vi "Do Transition.vi"(5 "VolatusAPI":refnum<class "VolatusAPI.lvclass">, 6 "State Loop Data in":T1, 7 "State Control":T9, 9 "Seq Name":string, 10 "Met Conditions":refnum<class "Condition.lvclass">[](array[class]), 11 "State in":refnum<class "State.lvclass">) -> (3 "State out":refnum<class "State.lvclass">, 4 "State Loop Data":T1)   [LabVIEW 2023, in "VolatusSeq.lvlib" / "State.lvclass"]
uses:
  State.lvclass
  State Control.ctl
  Sequence Time.ctl
  Variables/Variables.lvclass
  State Loop Data.ctl
  Iteration Actions/Iteration Actions.lvclass
  Command.ctl
  VolatusSeqConfig/Command Type.ctl
  messages/CmdDigital/Data.ctl
  messages/CmdAnalog/Data.ctl
  Send Type.ctl
  Volatus/VolatusAPI/VolatusAPI.lvclass
  Condition/Condition.lvclass
  Iteration Actions/Iteration Actions.lvclass/Iteration Actions.ctl
  State.lvclass/State.ctl
  VolatusSeq.lvlib
  Transition/Transition.lvclass
  VolatusSeqConfig/VolatusSeqConfig.lvlib
  Volatus/MessageQ/MessageQ.lvclass
  messages/CmdDigital/CmdDigital.lvlib
  messages/CmdAnalog/CmdAnalog.lvlib
  lv-vecto/Vecto/Channel DBL/Channel DBL.lvclass
  Format String/Format String.lvclass
  VolatusSeqConfig/Debug Flags.ctl
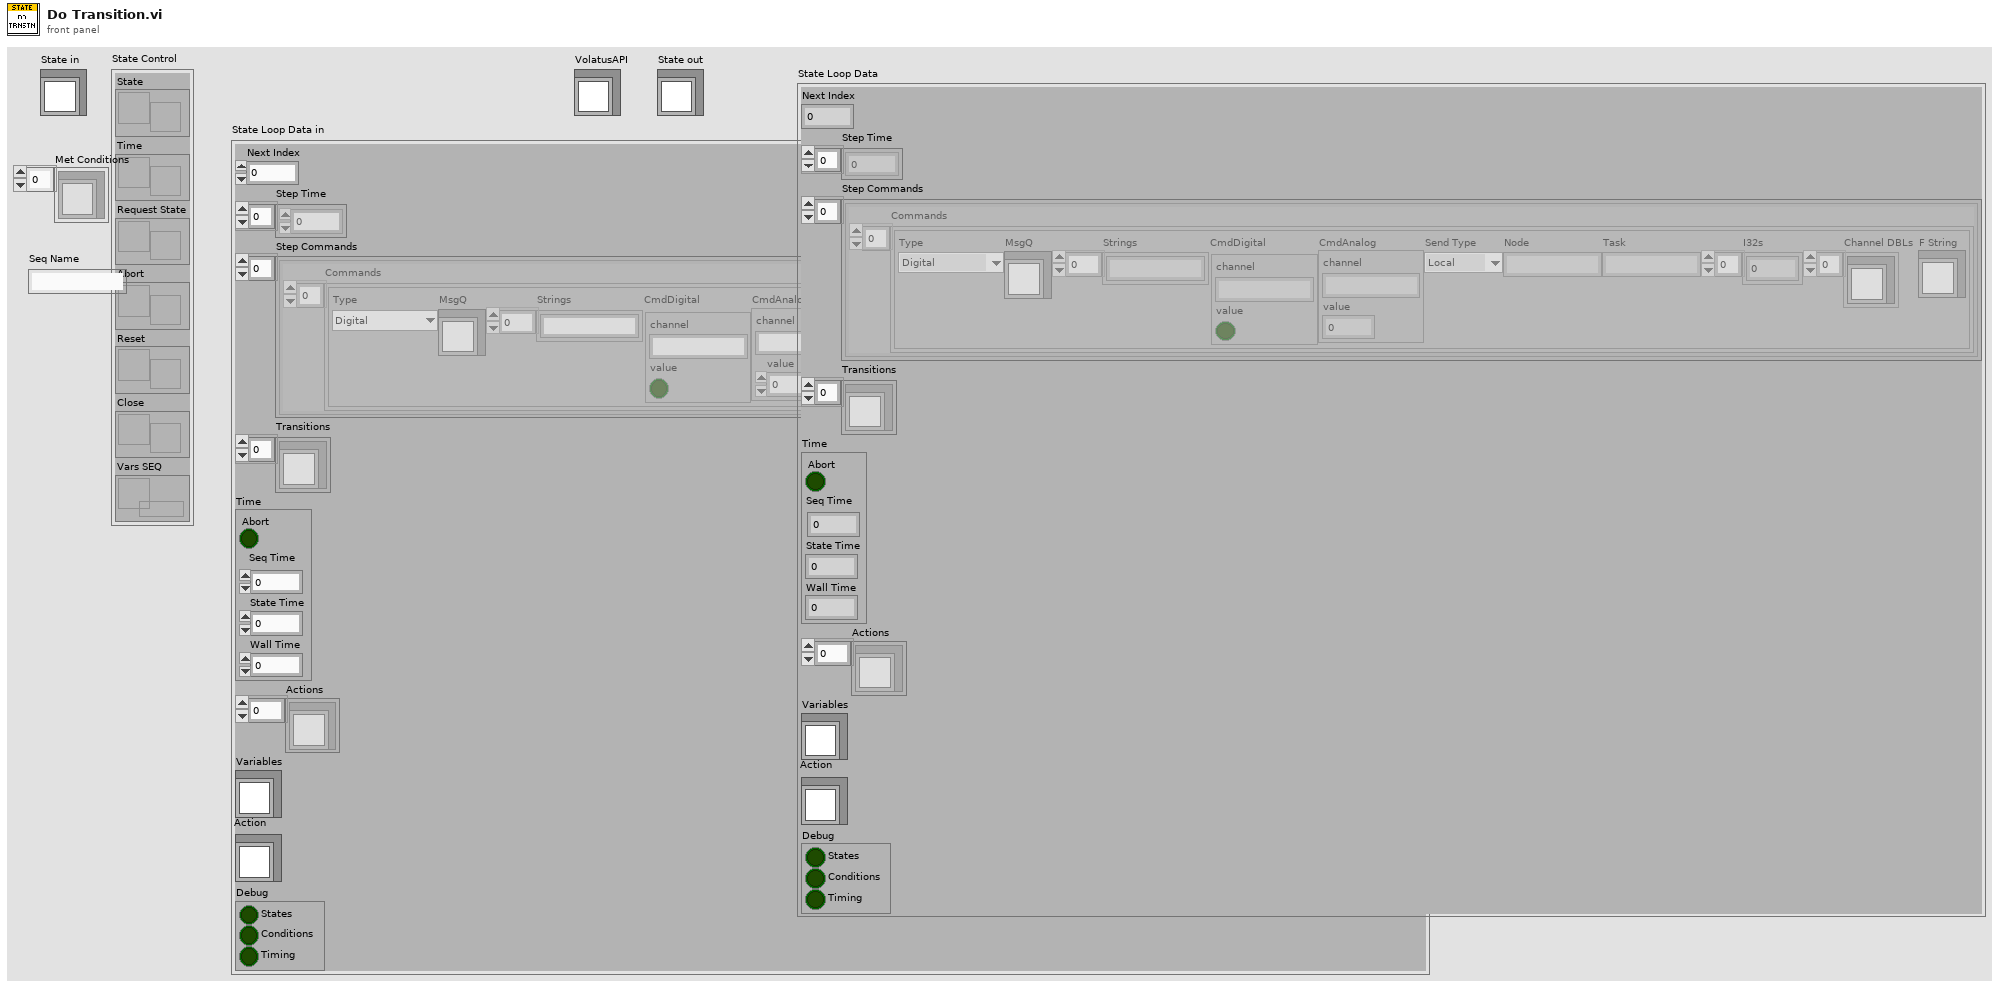
[diagram p1: front panel]
types:
  T1 = typedef "VolatusSeq.lvlib/State.lvclass/State Loop Data.ctl" = cluster{"Next Index":i32, "Step Time":dbl[], "Step Commands":cluster{"Commands":T2[]}[], "Transitions":refnum<class "Transition.lvclass">[], "Time":T7, "Actions":refnum<class "Iteration Actions.lvclass">[], "Variables":refnum<class "Variables.lvclass">, "Action":refnum<class "Iteration Actions.lvclass">, "Debug":T8}
  T2 = typedef "VolatusSeq.lvlib/Command.ctl" = cluster{"Type":T3, "MsgQ":refnum<class "MessageQ.lvclass">, "Strings":string[], "CmdDigital":T4, "CmdAnalog":T5, "Send Type":T6, "Node":string, "Task":string, "I32s":i32[], "Channel DBLs":refnum<class "Channel DBL.lvclass">[], "F String":refnum<class "Format String.lvclass">}
  T3 = typedef "VolatusSeqConfig.lvlib/Command Type.ctl" = enum16{"Digital", "Numeric", "Transition", "Stop", "StartLog", "StopLog", "Start", "Event", "Error", "HTTP", "ResetVar", "IncVar", "DecVar", "SaveVar", "LoadVar", "AddVar", "SubVar", "SetVar", "AddToVar"}
  T4 = typedef "CmdDigital.lvlib/Data.ctl" = cluster{"channel":string, "value":bool}
  T5 = typedef "CmdAnalog.lvlib/Data.ctl" = cluster{"channel":string, "value":dbl}
  T6 = typedef "VolatusSeq.lvlib/Send Type.ctl" = enum16{"Local", "Remote"}
  T7 = typedef "VolatusSeq.lvlib/Sequence Time.ctl" = cluster{"Abort":bool, "Seq Time":dbl, "State Time":dbl, "Wall Time":dbl}
  T8 = typedef "VolatusSeqConfig.lvlib/Debug Flags.ctl" = cluster{"States":bool, "Conditions":bool, "Timing":bool}
  T9 = typedef "VolatusSeq.lvlib/State Control.ctl" = cluster{"State":refnum<notifier>, "Time":refnum<notifier>, "Request State":refnum<notifier>, "Abort":refnum<notifier>, "Reset":refnum<notifier>, "Close":refnum<notifier>, "Vars SEQ":refnum<queue>}
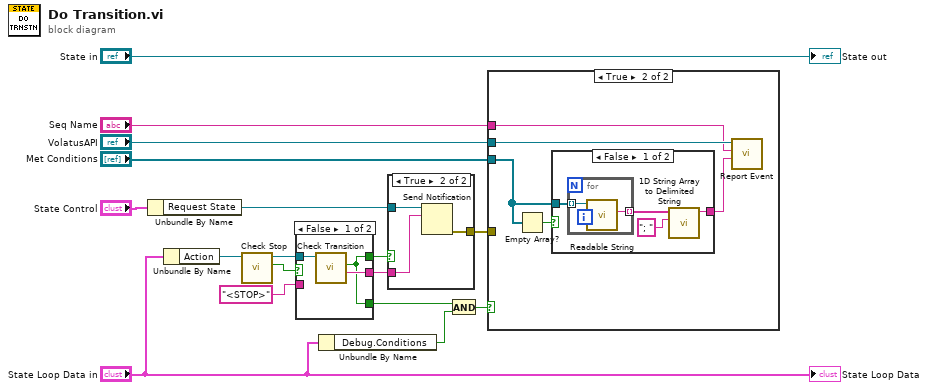
[diagram p0: block diagram]
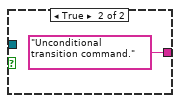
[diagram p3: hidden frame]
diagram:
  n1 = Unbundle By Name("State Control") -> ("Request State"=w13:refnum<notifier>)
  n2 = Unbundle By Name("State Loop Data in") -> ("Action"=w16:refnum<class "Iteration Actions.lvclass">)
  n3 = call "Check Stop.vi"("Iteration Actions in"=w16) -> ("Stop Seq"=w11:bool, "Iteration Actions out"=w12:refnum<class "Iteration Actions.lvclass">)  [unwired: 8 in, 1 out]
  n4 = case shown="False" w11 {
    selector: w11 -> [_ w22]
    tunnel: [w18 w22] -> w15
    tunnel: [w20 w21] -> w10
    tunnel: w12 -> [w19 _]
    tunnel: "<STOP>" ("Next State") -> [_ w21]
    tunnel: [w18 _] -> w7
    frame False {
      n5 = call "Check Transition.vi"("Iteration Actions in"=w19) -> ("Next State"=w20:string, "Transition"=w18:bool)  [unwired: 7 in, 2 out]
    }
    frame True {
    }
  }
  n6 = Unbundle By Name("State Loop Data in") -> ("Debug.Conditions"=w6:bool)
  n7 = case shown="True" w15 {
    tunnel: w10 -> [_ w24]
    tunnel: w13 -> [_ w25]
    tunnel: [_ w23] -> w2
    frame False {
    }
    frame True {
      n8 = Send Notification(notification=w24, notifier=w25) -> (error out=w23:errorcluster)  [unwired: 1 in, 1 out]
    }
  }
  n9 = And(x=w7, y=w6) -> (x .and. y?=w5:bool)
  n10 = case shown="True" w5 {
    tunnel: "VolatusAPI" -> [_ w30]
    tunnel: "Seq Name" -> [_ w29]
    tunnel: "Met Conditions" -> [_ w27]
    tunnel: w2 -> [_ _]
    frame False {
    }
    frame True {
      n11 = Empty Array?(array=w27) -> (empty?=w26:bool)
      n12 = case shown="False" w26 {
        tunnel: [w32 "Unconditional transition command." ("delimited string")] -> w28
        tunnel: w27 -> [w31 _]
        frame False {
          n13 = for {
            tunnel: w31 -> [w36] mode=indexing
            tunnel: [w35] -> w34 mode=indexing
            n14 = call-dynamic "Readable String.vi"("Condition in"=w36) -> ("String"=w35:string)  [unwired: 10 in]
          }
          n15 = call <vilib>:"1D String Array to Delimited String.vi"("delimiter"="; ", "string array"=w34) -> ("delimited string"=w32:string)  [unwired: 9 in]
        }
        frame True {
        }
      }
      n16 = call "Report Event.vi"("Message"=w28, "Context"=w29, "VolatusAPI in"=w30) -> ()  [unwired: 7 in, 2 out]
    }
  }
  "State out" <- "State in"
  "State Loop Data" <- "State Loop Data in"
